vi "Initialize Weather Station.vi"(8 "에러 입력(에러 없음)":errorcluster) -> (0 "에러 출력":errorcluster, 3 "파일 참조 번호":refnum<file>, 5 "날씨 데이터":T1)   [LabVIEW 2010]
doc: "이 VI는 기상 관측기 프로젝트의 일부입니다. 기상 데이터 클러스터를 생성하고 텍스트 파일 (Weather.txt)를 생성합니다. 기상 데이터 클러스터를 나타내는 헤더를 파일에 씁니다.\n\n입력: 에러 입력\n출력: 파일 참조 번호, 기상 데이터 클러스터, 에러 출력"
uses:
  <vilib>/Utility/file.llb/Application Directory.vi
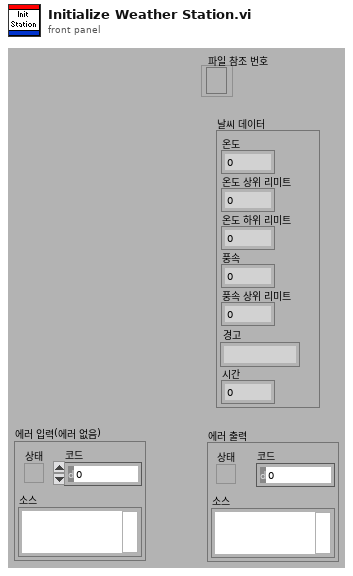
[diagram p1: front panel]
types:
  T1 = cluster{"온도":dbl, "온도 상위 리미트":dbl, "온도 하위 리미트":dbl, "풍속":dbl, "풍속 상위 리미트":dbl, "경고":string, "시간":dbl}
  T2 = enum16{"open", "replace", "create", "open or create", "replace or create", "replace or create with confirmation"}
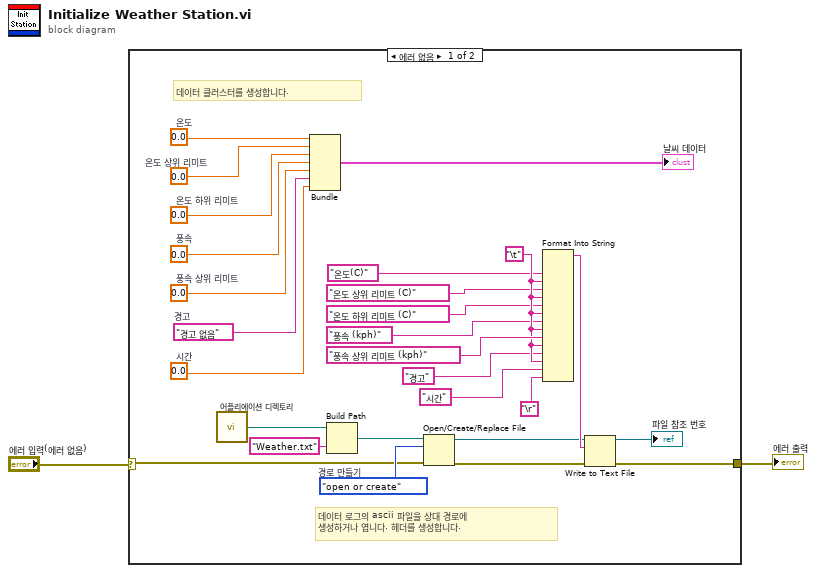
[diagram p0: block diagram]
diagram:
  n1 = case shown="에러 없음" "에러 입력(에러 없음)" {
    selector: "에러 입력(에러 없음)" -> [w6 w30]
    tunnel: [w28 w30] -> w2
    frame No Error {
      w4 = 0.0  # 시간
      w3 = 0.0  # 풍속 상위 리미트
      w12 = 0.0  # 풍속
      w7 = 0.0  # 온도 하위 리미트
      w8 = 0.0  # 온도 상위 리미트
      w9 = 0.0  # 온도
      w22 = "\t"
      w11 = "경고 없음"  # 경고
      # "데이터 로그의 ascii 파일을 상대 경로에 \n생성하거나 엽니다. 헤더를 생성합니다."
      # "데이터 클러스터를 생성합니다."
      n2 = call "어플리에이션 디렉토리"() -> ("Application Directory"=w5:path)
      n3 = Bundle("온도"=w9, "온도 상위 리미트"=w8, "온도 하위 리미트"=w7, "풍속"=w12, "풍속 상위 리미트"=w3, "경고"=w11, "시간"=w4) -> (→"날씨 데이터":T1)  [unwired: 1 in]
      n4 = Build Path "경로 만들기"(base path=w5, name or relative path="Weather.txt") -> (appended path=w14:path)
      n5 = Open/Create/Replace File(file path (use dialog)=w14, error in=w6, operation (0:open)=T2."open or create") -> (refnum out=w25:refnum<file>, error out=w27:errorcluster)  [unwired: 3 in, 1 out]
      n6 = Format Into String("온도(C)", w22, "온도 상위 리미트 (C)", w22, "온도 하위 리미트 (C)", w22, "풍속 (kph)", w22, "풍속 상위 리미트 (kph)", w22, "경고", w22, "시간", "\r") -> (resulting string=w29:string)  [unwired: 3 in, 1 out]
      n7 = Write to Text File(file (use dialog)=w25, text=w29, error in=w27) -> (refnum out=→"파일 참조 번호":refnum<file>, error out=w28:errorcluster)  [unwired: 1 in, 1 out]
    }
    frame Error {
    }
  }
  "에러 출력" <- w2
